vi "MSScript_Act_GetExpressions.vi"(8 "error in (no error)":errorcluster, 11 "MSScript in":refnum<class "MSScript.lvclass">) -> (0 "error out":errorcluster, 3 "MSScript out":refnum<class "MSScript.lvclass">)   [LabVIEW 2018, in "MSScript.lvclass"]
uses:
  MSScript.lvclass
  MSScript.lvclass/MSScript.ctl
  MSScript_Error_(6002)UndefinedSentence.vi
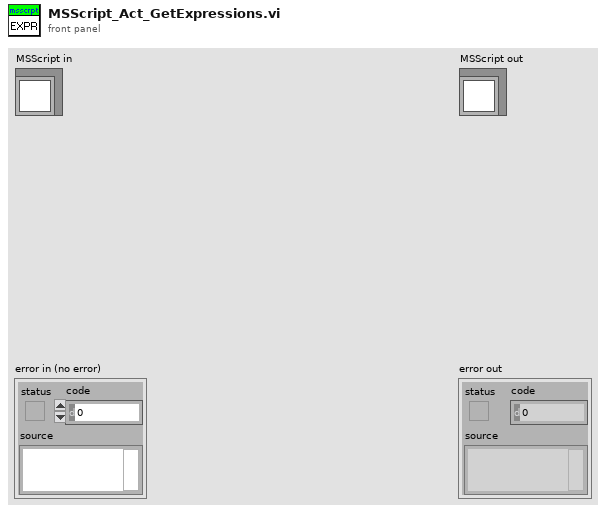
[diagram p1: front panel]
types:
  T1 = cluster{"Colour":u32, "Italic":bool, "Bold":bool}
  T2 = cluster{"Type":string, "NAME":cluster{"STR":string, "Start":i32}, "PARAMs":cluster{"STR":string, "Start":i32}[]}
  T3 = cluster{"Type":string, "NAME":cluster{"STR":string, "Start":i32}, "PARAMs":cluster{"STR":string, "Start":i32}[]}[]
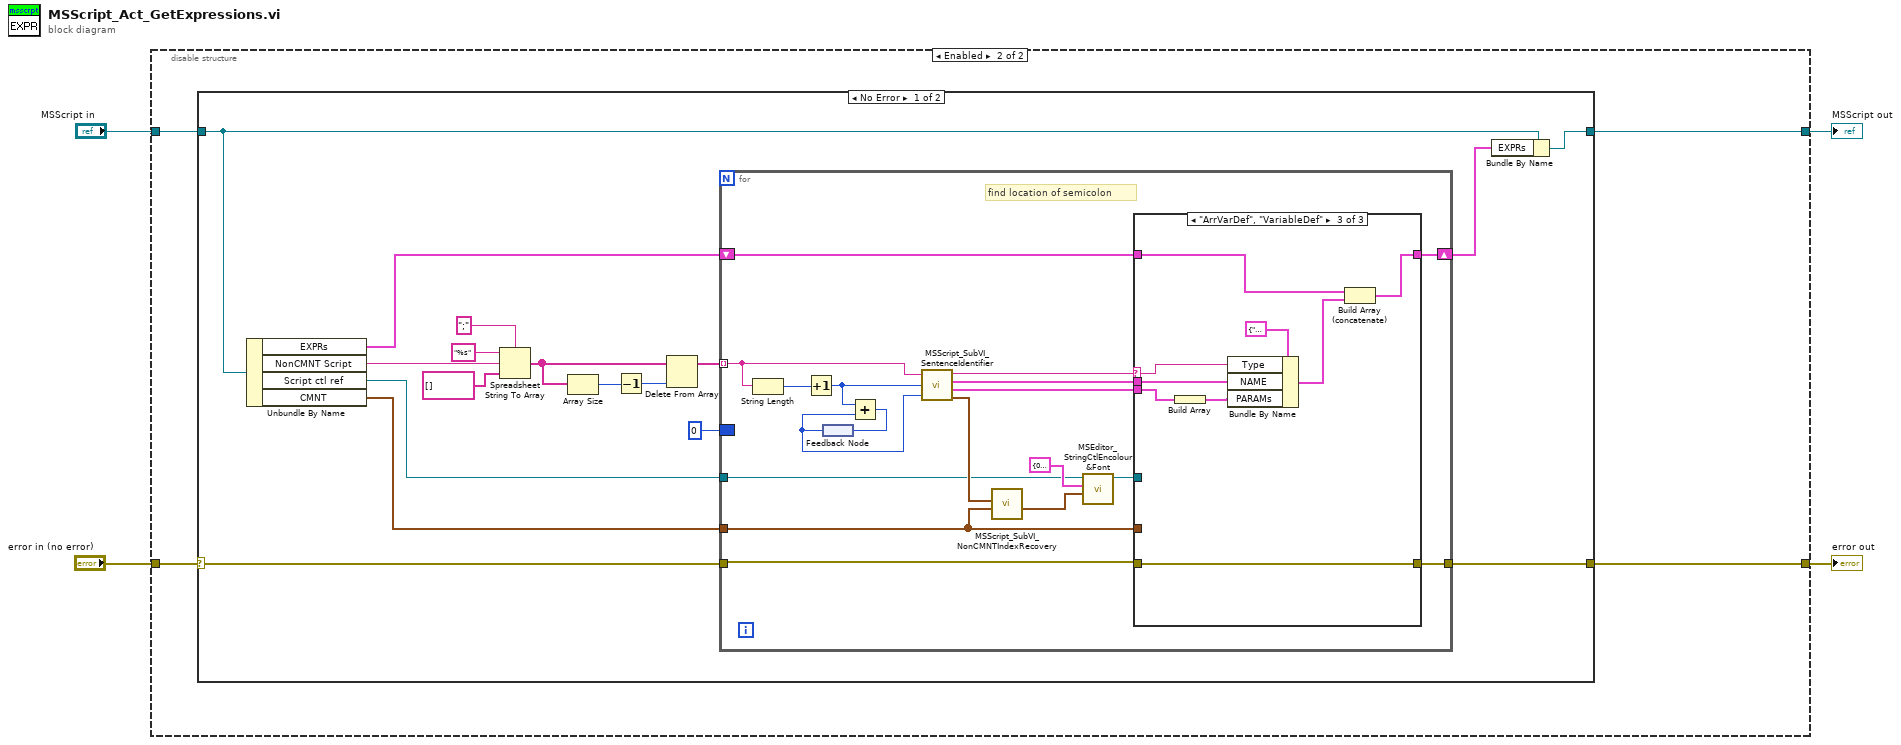
[diagram p0: block diagram]
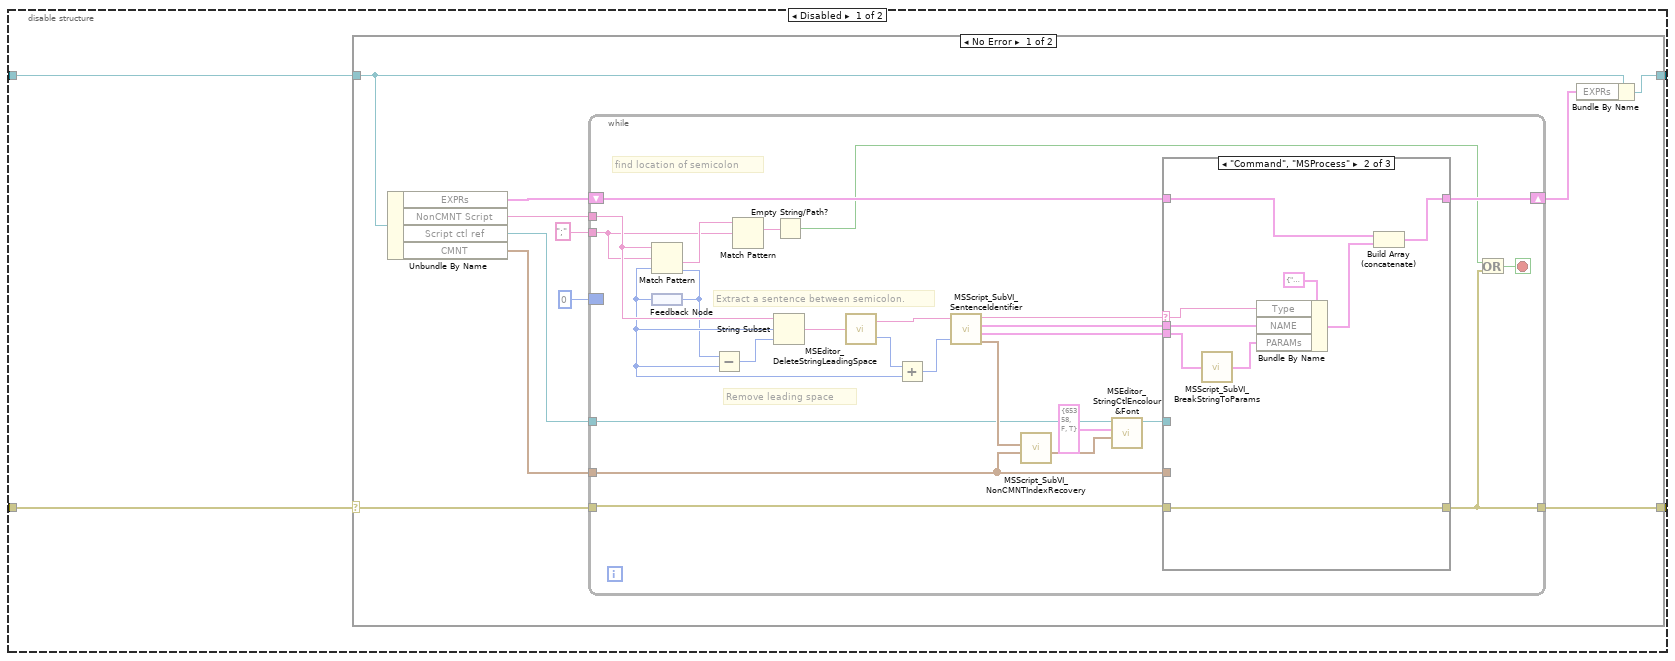
[diagram p2: hidden frame]
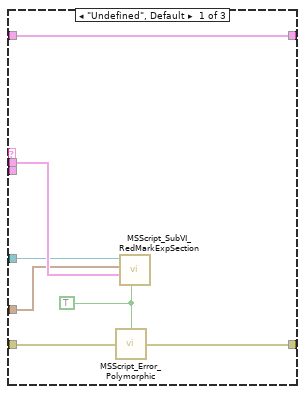
[diagram p3: hidden frame]
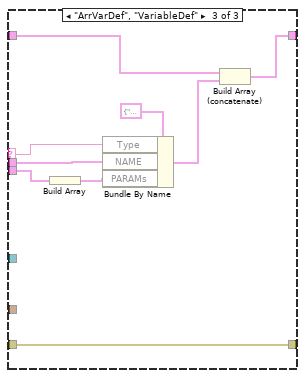
[diagram p4: hidden frame]
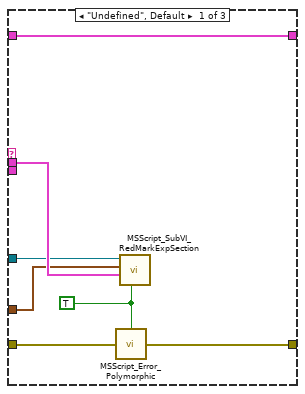
[diagram p6: hidden frame]
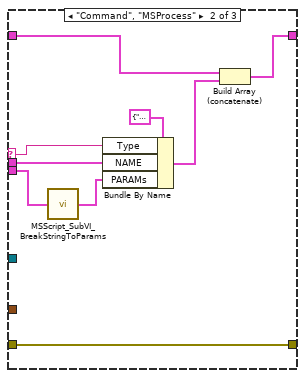
[diagram p7: hidden frame]
diagram:
  n1 = disable-structure shown="Enabled" {
    disable-tunnel: "error in (no error)" -> [w8 w75]
    disable-tunnel: [w7 w74] -> w3
    disable-tunnel: "MSScript in" -> [w6 w76]
    disable-tunnel: [w5 w73] -> w1
    frame Disabled {
      n2 = case shown="No Error" w8 {
        selector: w8 -> [w16 w72]
        tunnel: [w13 w72] -> w7
        tunnel: [w11 w71] -> w5
        tunnel: w6 -> [w14 w71]
        frame No Error {
          n3 = Unbundle By Name(w14) -> ("EXPRs"=w12:T3, "NonCMNT Script"=w19:string, "Script ctl ref"=w17:refnum<vi>, "CMNT"=w15:cluster{"Start":u32, "End":u32}[])
          n4 = while {
            tunnel: w19 -> [w44]
            tunnel: w17 -> [w33]
            tunnel: w16 -> [w32]
            tunnel: [w22] -> w13
            tunnel: w15 -> [w25]
            shift-right: [w29] -> w10
            shift-left: w12 -> [w30]
            border: 0 -> [_]
            tunnel: ";" -> [w21]
            stop <- w24 stop-if-true
            # "Extract a sentence between semicolon."
            # "Remove leading space"
            # "find location of semicolon"
            n5 = feedback #1() -> (w39:i32)
            n6 = Match Pattern(string=w44, regular expression=w21, offset (0)=w39) -> (after substring=w42:string, offset past match=w20:i32)  [unwired: 2 out]
            n7 = feedback-in #1(w20) -> ()
            n8 = Subtract(x=w20, y=w39) -> (x-y=w43:i32)
            n9 = Match Pattern(string=w42, regular expression=w21) -> (match substring=w45:string)  [unwired: 1 in, 3 out]
            n10 = String Subset(string=w44, offset (0)=w39, length (rest)=w43) -> (substring=w41:string)
            n11 = Empty String/Path?(string/path=w45) -> (empty?=w23:bool)
            n12 = call "MSEditor_DeleteStringLeadingSpace.vi"("string in"=w41) -> ("string after leading space"=w38:string, "offset past leading space"=w40:i32)
            n13 = Add(x=w40, y=w39) -> (x+y=w37:i32)
            n14 = call "MSScript_SubVI_SentenceIdentifier.vi"("IniPosition"=w37, "Single sentance in"=w38) -> ("Delimiter SELs"=w35:cluster{"Start":u32, "End":u32}[], "Parameter string"=w26:cluster{"Str":string, "Start":i32}, "Name string"=w27:cluster{"Str":string, "Start":i32}, "Sentence type"=w28:string)  [unwired: 2 in]
            n15 = call "MSScript_SubVI_NonCMNTIndexRecovery.vi"("SEL of CMNT"=w25, "NonCMNT.SEL"=w35) -> ("RecoverySEL"=w34:cluster{"Start":u32, "End":u32}[])  [unwired: 5 in]
            n16 = call "MSEditor_StringCtlEncolour&Font.vi"("SELs"=w34, "TextProperties"=T1 {"Colour"=65358, "Italic"=FALSE, "Bold"=TRUE}, "String ctl ref"=w33) -> ("String ctl ref out"=w31:refnum<vi>)  [unwired: 7 in, 1 out]
            n17 = case shown="\"Command\", \"MSProcess\"" w28 {
              selector: w28 -> [_ w54 w68]
              tunnel: w27 -> [w49 w53 w67]
              tunnel: w26 -> [_ w61 w66]
              tunnel: w31 -> [w48 _ _]
              tunnel: w25 -> [w47 _ _]
              tunnel: w32 -> [w51 w60 w70]
              tunnel: [w50 w60 w70] -> w22
              tunnel: w30 -> [w52 w59 w62]
              tunnel: [w52 w57 w63] -> w29
              frame "Undefined", Default {
                w46 = TRUE ("ErrBoolean")
                n18 = call-poly "MSScript_Error_Polymorphic.vi"("error in (no error)"=w51, "ErrBoolean"=w46) -> ("error out"=w50:errorcluster)
                n19 = call "MSScript_SubVI_RedMarkExpSection.vi"("Enable"=w46, "Expression.Section"=w49, "CMNT"=w47, "String in"=w48) -> ()  [unwired: 8 in]
              }
              frame "Command", "MSProcess" {
                n20 = call "MSScript_SubVI_BreakStringToParams.vi"("string"=w61) -> ("PARAMs"=w56:cluster{"Str":string, "Start":i32}[])
                n21 = Bundle By Name(cluster=T2 {"Type"="", "NAME"={"STR"="", "Start"=0}, "PARAMs"=[]} ("Expression"), "Type"=w54, "NAME"=w53, "PARAMs"=w56) -> (w55:T2)
                n22 = Build Array (concatenate)(w59, w55) -> (w57:T3)
              }
              frame "ArrVarDef", "VariableDef" {
                n23 = Build Array(w66) -> (w65:cluster{"Str":string, "Start":i32}[])
                n24 = Bundle By Name(cluster=T2 {"Type"="", "NAME"={"STR"="", "Start"=0}, "PARAMs"=[]} ("Expression"), "Type"=w68, "NAME"=w67, "PARAMs"=w65) -> (w64:T2)
                n25 = Build Array (concatenate)(w62, w64) -> (w63:T3)
              }
            }
            n26 = Or(x=w23, y=w22) -> (x .or. y?=w24:bool)
          }
          n27 = Bundle By Name(cluster=w14, "EXPRs"=w10) -> (w11:refnum<class "MSScript.lvclass">)
        }
        frame Error {
        }
      }
    }
    frame Enabled {
      n28 = case shown="No Error" w75 {
        selector: w75 -> [w91 w138]
        tunnel: [w88 w138] -> w74
        tunnel: [w86 w137] -> w73
        tunnel: w76 -> [w89 w137]
        frame No Error {
          n29 = Unbundle By Name(w89) -> ("EXPRs"=w87:T3, "NonCMNT Script"=w81:string, "Script ctl ref"=w92:refnum<vi>, "CMNT"=w90:cluster{"Start":u32, "End":u32}[])
          n30 = Spreadsheet String To Array(delimiter (Tab)=";", format string="%s", spreadsheet string=w81, array type (2D Dbl)=string[] []) -> (array=w80:string[])
          n31 = Array Size(array=w80) -> (size(s)=w78:i32)
          n32 = Decrement(x=w78) -> (x-1=w77:i32)
          n33 = Delete From Array(array=w80, index=w77) -> (array with subset deleted=w79:string[])  [unwired: 1 in, 1 out]
          n34 = for {
            tunnel: w92 -> [w108]
            tunnel: w91 -> [w107]
            tunnel: [w99] -> w88
            tunnel: w90 -> [w100]
            shift-right: [w104] -> w85
            shift-left: w87 -> [w105]
            border: 0 -> [_]
            tunnel: w79 -> [w94] mode=indexing
            # "find location of semicolon"
            n35 = String Length(string=w94) -> (length=w98:i32)
            n36 = Increment(x=w98) -> (x+1=w95:i32)
            n37 = feedback #2() -> (w96:i32)
            n38 = Add(x=w95, y=w96) -> (x+y=w97:i32)
            n39 = feedback-in #2(w97) -> ()
            n40 = call "MSScript_SubVI_SentenceIdentifier.vi"("IniPosition"=w96, "strlen"=w95, "Single sentance in"=w94) -> ("Delimiter SELs"=w110:cluster{"Start":u32, "End":u32}[], "Parameter string"=w101:cluster{"Str":string, "Start":i32}, "Name string"=w102:cluster{"Str":string, "Start":i32}, "Sentence type"=w103:string)  [unwired: 1 in]
            n41 = call "MSScript_SubVI_NonCMNTIndexRecovery.vi"("SEL of CMNT"=w100, "NonCMNT.SEL"=w110) -> ("RecoverySEL"=w109:cluster{"Start":u32, "End":u32}[])  [unwired: 5 in]
            n42 = call "MSEditor_StringCtlEncolour&Font.vi"("SELs"=w109, "TextProperties"=T1 {"Colour"=0, "Italic"=FALSE, "Bold"=TRUE}, "String ctl ref"=w108) -> ("String ctl ref out"=w106:refnum<vi>)  [unwired: 7 in, 1 out]
            n43 = case shown="\"ArrVarDef\", \"VariableDef\"" w103 {
              selector: w103 -> [_ w120 w134]
              tunnel: w102 -> [w115 w119 w133]
              tunnel: w101 -> [_ w127 w132]
              tunnel: w106 -> [w114 _ _]
              tunnel: w100 -> [w113 _ _]
              tunnel: w107 -> [w117 w126 w136]
              tunnel: [w116 w126 w136] -> w99
              tunnel: w105 -> [w118 w125 w128]
              tunnel: [w118 w123 w129] -> w104
              frame "Undefined", Default {
                w112 = TRUE ("ErrBoolean")
                n44 = call-poly "MSScript_Error_Polymorphic.vi"("error in (no error)"=w117, "ErrBoolean"=w112) -> ("error out"=w116:errorcluster)
                n45 = call "MSScript_SubVI_RedMarkExpSection.vi"("Enable"=w112, "Expression.Section"=w115, "CMNT"=w113, "String in"=w114) -> ()  [unwired: 8 in]
              }
              frame "Command", "MSProcess" {
                n46 = call "MSScript_SubVI_BreakStringToParams.vi"("string"=w127) -> ("PARAMs"=w122:cluster{"Str":string, "Start":i32}[])
                n47 = Bundle By Name(cluster=T2 {"Type"="", "NAME"={"STR"="", "Start"=0}, "PARAMs"=[]} ("Expression"), "Type"=w120, "NAME"=w119, "PARAMs"=w122) -> (w121:T2)
                n48 = Build Array (concatenate)(w125, w121) -> (w123:T3)
              }
              frame "ArrVarDef", "VariableDef" {
                n49 = Build Array(w132) -> (w131:cluster{"Str":string, "Start":i32}[])
                n50 = Bundle By Name(cluster=T2 {"Type"="", "NAME"={"STR"="", "Start"=0}, "PARAMs"=[]} ("Expression"), "Type"=w134, "NAME"=w133, "PARAMs"=w131) -> (w130:T2)
                n51 = Build Array (concatenate)(w128, w130) -> (w129:T3)
              }
            }
          }
          n52 = Bundle By Name(cluster=w89, "EXPRs"=w85) -> (w86:refnum<class "MSScript.lvclass">)
        }
        frame Error {
        }
      }
    }
  }
  "error out" <- w3
  "MSScript out" <- w1
